vi "ifft_cp_alamouti.vi"(8 "CP Length":u32, 9 "FFT Size":u32, 11 "Modulated Stream":cdb[](array[numeric])) -> (3 "Baseband Streams":cdb[][](array[numeric]))   [LabVIEW 2014]
uses:
  <vilib>/Analysis/2dsp.llb/Inverse Complex FFT.vi
  <vilib>/Analysis/NI_AALPro.lvlib
panel:
  out "Stream + CP":cdb[](array[numeric])
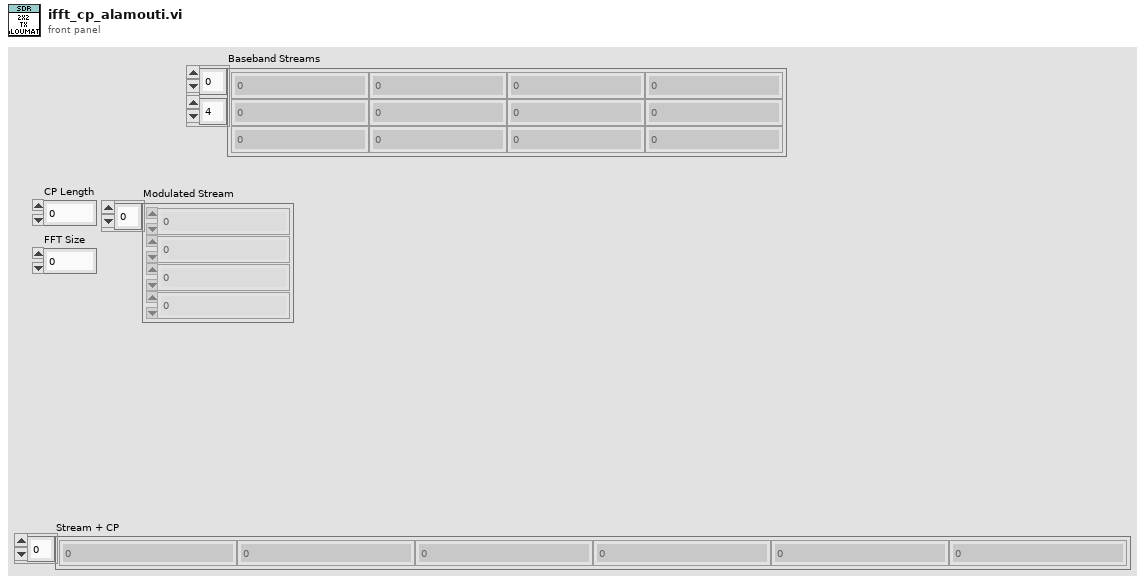
[diagram p1: front panel]
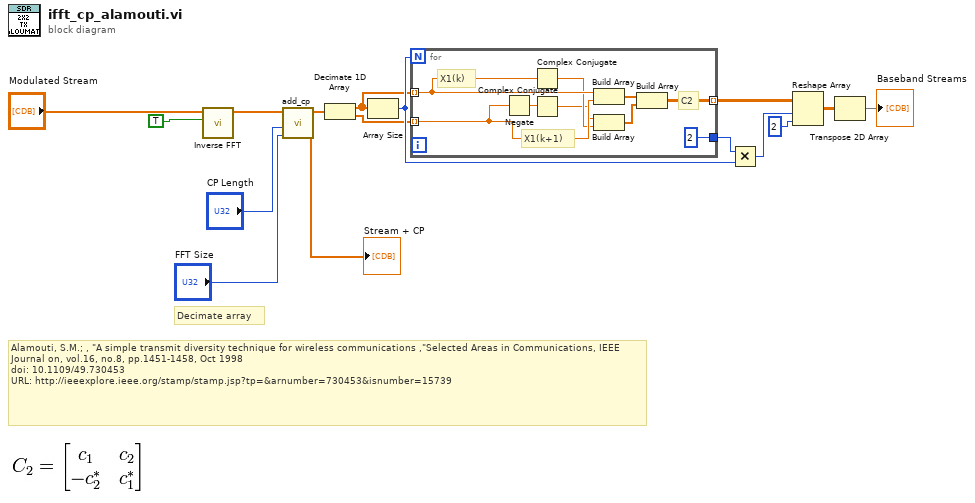
[diagram p0: block diagram]
diagram:
  # "Decimate array"
  # "Alamouti, S.M.; , \"A simple transmit diversity technique for wireless communications ,\"Selected Areas in Communications, IEEE Journal on, vol.16, no.8, pp.1451-1458, Oct 1998 \ndoi: 10.1109/49.730453\nURL: http://ieeexplore.ieee.org/stamp/stamp.jsp?tp=&arnumber=730453&isnumber=15739"
  n1 = call-poly <vilib>:"Inverse FFT.vi"("shift?"=TRUE, "FFT {X}"="Modulated Stream") -> ("X"=w8:cdb[])  [unwired: 8 in, 1 out]
  n2 = call "add_cp.vi"("FFT size"="FFT Size", "CP length"="CP Length", "time_samples"=w8) -> ("cp ofdm symbol"=w3:cdb[])  [unwired: 8 in]
  "Stream + CP" <- w3
  n3 = Decimate 1D Array(w3) -> (w1:cdb[], w2:cdb[])
  n4 = Array Size(array=w1) -> (size(s)=w4:i32)
  n5 = for {
    N: w4 -> [_]
    tunnel: [2 ("x")] -> w14
    tunnel: [w23] -> w12 mode=indexing
    tunnel: w1 -> [w20] mode=indexing
    tunnel: w2 -> [w19] mode=indexing
    # "C2"
    # "X1(k)"
    # "X1(k+1)"
    n6 = Negate(x=w19) -> (-x=w18:cdb)
    n7 = Complex Conjugate(1:w20) -> (0:w17:cdb)
    n8 = Complex Conjugate(1:w18) -> (0:w16:cdb)
    n9 = Build Array(w20, w19) -> (w22:cdb[])
    n10 = Build Array(w16, w17) -> (w21:cdb[])
    n11 = Build Array(w22, w21) -> (w23:cdb[][])
  }
  n12 = Multiply(x=w14, y=w4) -> (x*y=w11:i32)
  n13 = Reshape Array(w12, w11, 2 ("dimension size")) -> (w15:cdb[][])
  n14 = Transpose 2D Array(2D array=w15) -> (transposed array=→"Baseband Streams":cdb[][])
